vi "Set_Oscilloscope.vi"(8 "error in (no error)":errorcluster, 11 "Control-Server in":refnum<class "Control-Server.lvclass">) -> (0 "error out":errorcluster, 3 "Control-Server out":refnum<class "Control-Server.lvclass">)   [LabVIEW 2015, in "Control-Server.lvclass"]
uses:
  Control-Server.lvclass
  Config/config_names_def.ctl
  dependecies/ControlsVIs/Clusters-def/Message types.ctl
  Message/Message.lvclass
  Oscilloscope/TELEDINE_LECROY/TELEDINE_LECROY.lvclass
  Control-Server.lvclass/Control-Server.ctl
  Message/Message.lvclass/Message.ctl
  GeneralFunctionality/GeneralFunctionality.lvclass/GeneralFunctionality.ctl
  Detector/Detector.lvclass
  Config/Config.lvclass
  GeneralFunctionality/GeneralFunctionality.lvclass
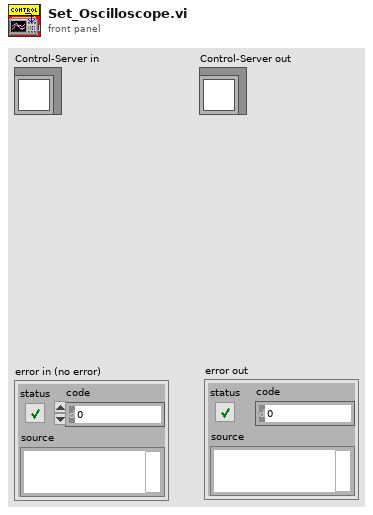
[diagram p1: front panel]
types:
  T1 = typedef "Message types.ctl" = string
  T2 = typedef "Config.lvclass/config_names_def.ctl" = string
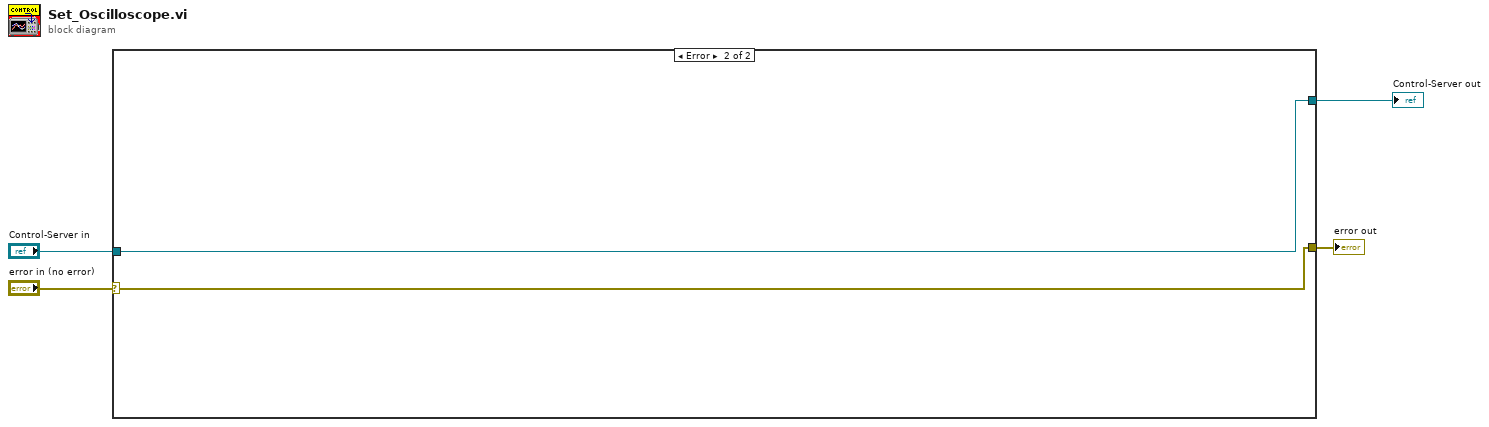
[diagram p0: block diagram]
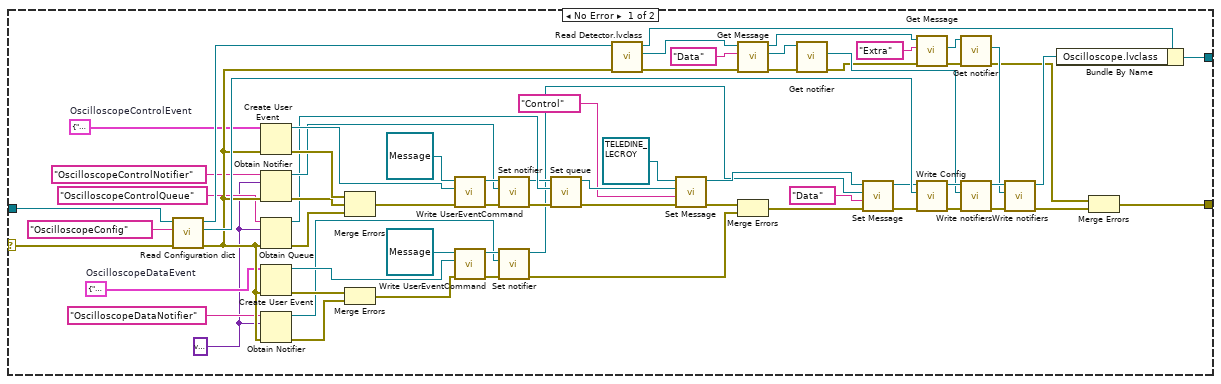
[diagram p2: hidden frame]
diagram:
  n1 = case shown="Error" "error in (no error)" {
    selector: "error in (no error)" -> [w5 w72]
    tunnel: [w67 w71] -> w4
    tunnel: [w66 w72] -> w3
    tunnel: "Control-Server in" -> [w65 w71]
    frame No Error {
      w57 = cluster{"command":string, "data":variant} {"command"="", "data"=variant}  # OscilloscopeControlEvent
      w24 = variant
      w51 = cluster{"command":string, "data":variant} {"command"="", "data"=variant}  # OscilloscopeDataEvent
      n2 = call "Read Configuration dict.vi"("error in (no error)"=w5, "Config Name"=T2 "OscilloscopeConfig", "Control in"=w65) -> ("error out"=w64:errorcluster, "Config"=w70:refnum<class "Config.lvclass">, "Control out"=w63:refnum<class "Control-Server.lvclass">)  [unwired: 6 in]
      n3 = Create User Event(user event datatype=w57, error in=w64) -> (user event=w59:refnum<user-event>, error out=w55:errorcluster)
      n4 = Obtain Notifier(name (unnamed)="OscilloscopeControlNotifier" ("nom (aucun)"), notification data type=w24, error in (no error)=w64) -> (notifier out=w53:refnum<notifier>, error out=w54:errorcluster)  [unwired: 1 in, 1 out]
      n5 = Obtain Queue(name (unnamed)="OscilloscopeControlQueue", element data type=w24, error in (no error)=w64) -> (queue out=w39:refnum<queue>, error out=w38:errorcluster)  [unwired: 2 in, 1 out]
      n6 = Create User Event(user event datatype=w51, error in=w64) -> (user event=w48:refnum<user-event>, error out=w45:errorcluster)
      n7 = Obtain Notifier(name (unnamed)="OscilloscopeDataNotifier" ("nom (aucun)"), notification data type=w24, error in (no error)=w64) -> (notifier out=w43:refnum<notifier>, error out=w44:errorcluster)  [unwired: 1 in, 1 out]
      n8 = Merge Errors(w55, w54, w38) -> (w52:errorcluster)
      n9 = Merge Errors(w45, w44) -> (w42:errorcluster)
      n10 = call "Write UserEventCommand.vi"("error in (no error)"=w52, "UserEventCommand"=w59, "Message en entrée"=refnum<class "Message.lvclass"> refnum ("Message.lvclass")) -> ("error out"=w56:errorcluster, "Message en sortie"=w60:refnum<class "Message.lvclass">)  [unwired: 7 in]
      n11 = call "Write UserEventCommand.vi"("error in (no error)"=w42, "UserEventCommand"=w48, "Message en entrée"=refnum<class "Message.lvclass"> refnum ("Message.lvclass")) -> ("error out"=w46:errorcluster, "Message en sortie"=w47:refnum<class "Message.lvclass">)  [unwired: 7 in]
      n12 = call "Set notifier.vi"("error in (no error)"=w56, "notifier"=w53, "Message en entrée"=w60) -> ("error out"=w37:errorcluster, "Message en sortie"=w36:refnum<class "Message.lvclass">)  [unwired: 7 in]
      n13 = call "Set notifier.vi"("error in (no error)"=w46, "notifier"=w43, "Message en entrée"=w47) -> ("error out"=w41:errorcluster, "Message en sortie"=w29:refnum<class "Message.lvclass">)  [unwired: 7 in]
      n14 = call "Set queue.vi"("error in (no error)"=w37, "queue"=w39, "Message in"=w36) -> ("error out"=w25:errorcluster, "Message out"=w34:refnum<class "Message.lvclass">)  [unwired: 7 in]
      n15 = call "Read Detector.lvclass.vi"("error in (no error)"=w64, "Control in"=w63) -> ("error out"=w19:errorcluster, "Detector.lvclass"=w17:refnum<class "Detector.lvclass">, "Control out"=w62:refnum<class "Control-Server.lvclass">)  [unwired: 7 in]
      n16 = call "Set Message.vi"("error in (no error)"=w25, "Message type"=T1 "Control", "Message.lvclass"=w34, "GeneralFunctionality en entrée"=refnum<class "TELEDINE_LECROY.lvclass"> refnum ("TELEDINE_LECROY.lvclass")) -> ("error out"=w28:errorcluster, "GeneralFunctionality en sortie"=w32:refnum<class "TELEDINE_LECROY.lvclass">)  [unwired: 6 in]
      n17 = call "Get Message.vi"("error in (no error)"=w19, "Message type"=T1 "Data", "GeneralFunctionality en entrée"=w17) -> ("error out"=w18:errorcluster, "Message.lvclass"=w22:refnum<class "Message.lvclass">, "GeneralFunctionality en sortie"=w11:refnum<class "Detector.lvclass">)  [unwired: 6 in]
      n18 = Merge Errors(w28, w41) -> (w27:errorcluster)
      n19 = call "Get notifier.vi"("error in (no error)"=w18, "Message en entrée"=w22) -> ("error out"=w12:errorcluster, "notifier"=w21:refnum<notifier>)  [unwired: 7 in, 1 out]
      n20 = call "Set Message.vi"("error in (no error)"=w27, "Message type"=T1 "Data", "Message.lvclass"=w29, "GeneralFunctionality en entrée"=w32) -> ("error out"=w26:errorcluster, "GeneralFunctionality en sortie"=w31:refnum<class "TELEDINE_LECROY.lvclass">)  [unwired: 6 in]
      n21 = call "Get Message.vi"("error in (no error)"=w12, "Message type"=T1 "Extra", "GeneralFunctionality en entrée"=w11) -> ("error out"=w9:errorcluster, "Message.lvclass"=w8:refnum<class "Message.lvclass">)  [unwired: 6 in, 1 out]
      n22 = call "Write Config.vi"("error in (no error)"=w26, "Config.lvclass"=w70, "GeneralFunctionality en entrée"=w31) -> ("error out"=w20:errorcluster, "GeneralFunctionality en sortie"=w23:refnum<class "TELEDINE_LECROY.lvclass">)  [unwired: 7 in]
      n23 = call "Get notifier.vi"("error in (no error)"=w9, "Message en entrée"=w8) -> ("error out"=w6:errorcluster, "notifier"=w7:refnum<notifier>)  [unwired: 7 in, 1 out]
      n24 = call-dynamic "Write notifiers.vi"("error in (no error)"=w20, "notifier"=w21, "Oscilloscope in"=w23) -> ("error out"=w15:errorcluster, "Oscilloscope out"=w13:refnum<class "TELEDINE_LECROY.lvclass">)  [unwired: 7 in]
      n25 = call-dynamic "Write notifiers.vi"("error in (no error)"=w15, "notifier"=w7, "Oscilloscope in"=w13) -> ("error out"=w14:errorcluster, "Oscilloscope out"=w68:refnum<class "TELEDINE_LECROY.lvclass">)  [unwired: 7 in]
      n26 = Bundle By Name(cluster=w62, "Oscilloscope.lvclass"=w68) -> (w67:refnum<class "Control-Server.lvclass">)
      n27 = Merge Errors(w6, w14) -> (w66:errorcluster)
    }
    frame Error {
    }
  }
  "error out" <- w3
  "Control-Server out" <- w4
